vi "Dimostatore.vi"() -> ()   [LabVIEW 2019]
uses:
  ByteGSAPIBase.lvclass
  FetchCalibration/Converted_Slug_Cluster.ctl
  CalibrationMeasurements/BodyCalibrazioneMisure.ctl
  6d3d0a70-a223-4ddd-b0d3-7207305fe689.vi
  85eea304-0067-4311-882a-d02f57de18c2.vi
panel:
  out "Valore misurato":string
  out "Valore di riferimento":string
  in  "Start":bool
  in  "Send":bool
  out "Infobox":string
  out "Strumenti da calibrare":i32(listbox)
  in  "Exit":bool=TRUE
  in  "Calibrate":bool
  in  "error out":errorcluster
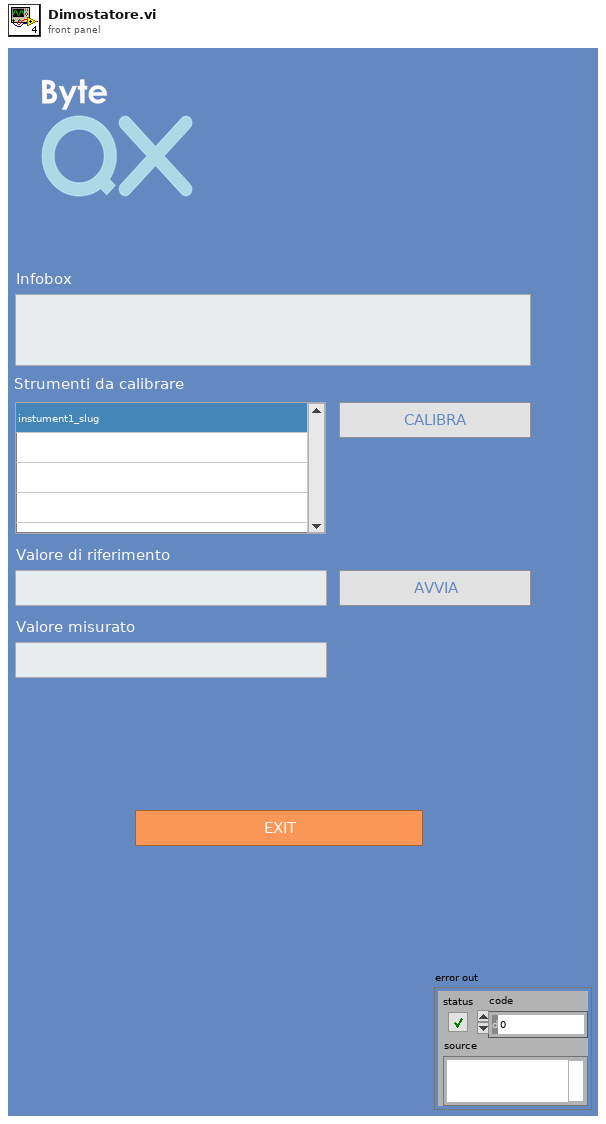
[diagram p1: front panel]
types:
  T1 = cluster{"nome":string, cluster{"Measurement_Id":i32, "Passed?":bool}[]}[]
  T2 = typedef "ByteGSWebAPI.lvlib/ByteGSAPIBase.lvclass/BodyCalibrazioneMisure.ctl" = cluster{"strumento_riferimento":cluster{"id":u16, "nome":string}, "controls":cluster{"id":u16, "descrizione":string, "numero_misure_necessarie":u16, "riferimento_obiettivo":dbl, "mpe_max":dbl, "mpe_min":dbl, "deviazione_standard":dbl, "incertezza":dbl}[], "temperatura_c":dbl, "umidita":dbl}
  T3 = typedef "ByteGSWebAPI.lvlib/ByteGSAPIBase.lvclass/Converted_Slug_Cluster.ctl" = cluster{"id":u32, "instrument":string, "name":string, "date":timestamp}
  T4 = cluster{"ByteGSAPIBase in":refnum<class "ByteGSAPIBase.lvclass">, "Expired_Instruments":T3[], "Calibrations":T2, "Strumenti_calibrati":cluster{"nome":string, cluster{"Measurement_Id":i32, "Passed?":bool}[]}[], "Instr_index":i32, "Calib_index":i32, "Instruments_Slug":string[]}
  T5 = cluster{"id":u16, "descrizione":string, "numero_misure_necessarie":u16, "riferimento_obiettivo":dbl, "mpe_max":dbl, "mpe_min":dbl, "deviazione_standard":dbl, "incertezza":dbl}[]
  T6 = cluster{"id":u16, "descrizione":string, "numero_misure_necessarie":u16, "riferimento_obiettivo":dbl, "mpe_max":dbl, "mpe_min":dbl, "deviazione_standard":dbl, "incertezza":dbl}
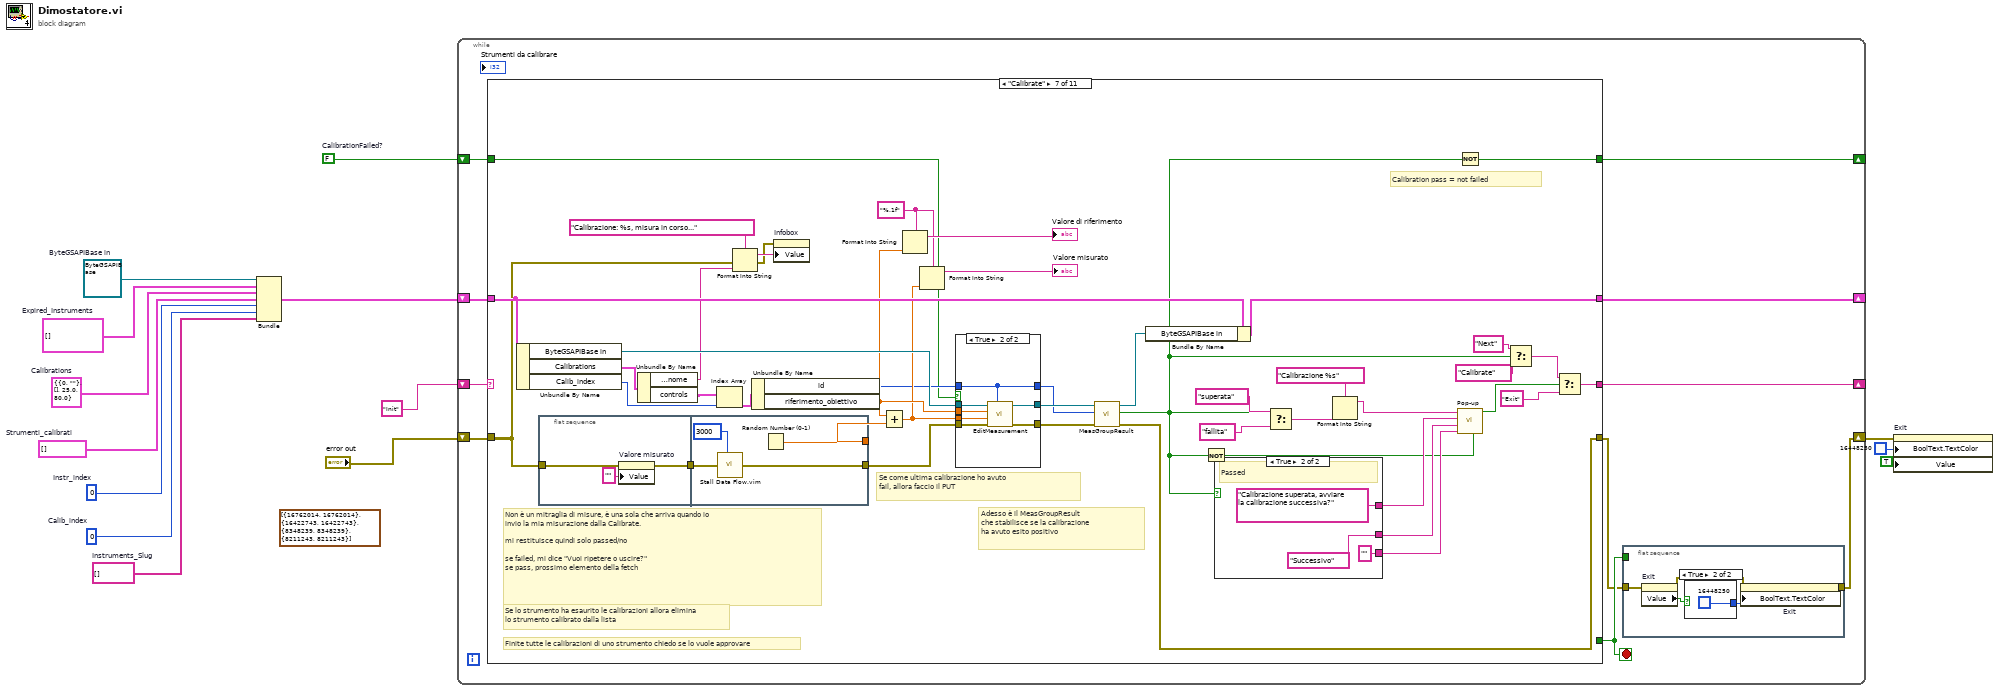
[diagram p0: block diagram]
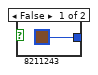
[diagram p2: hidden frame]
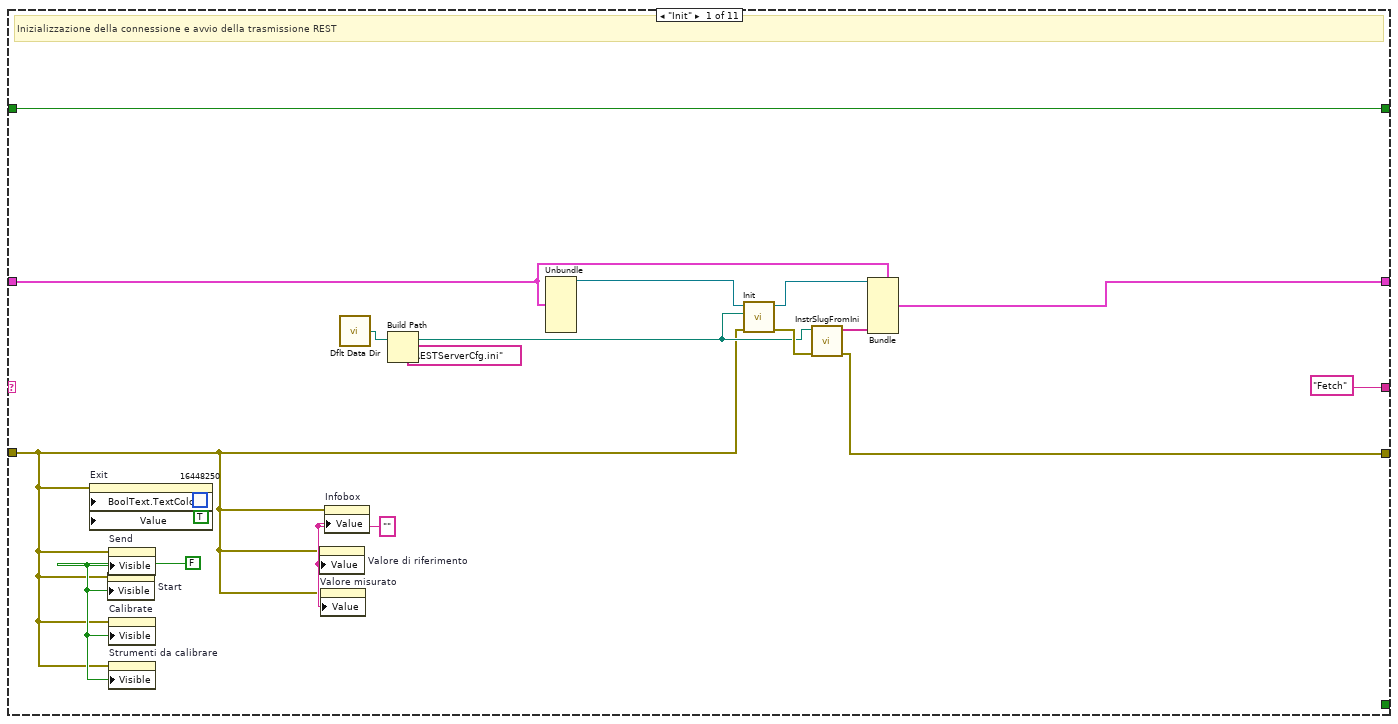
[diagram p3: hidden frame]
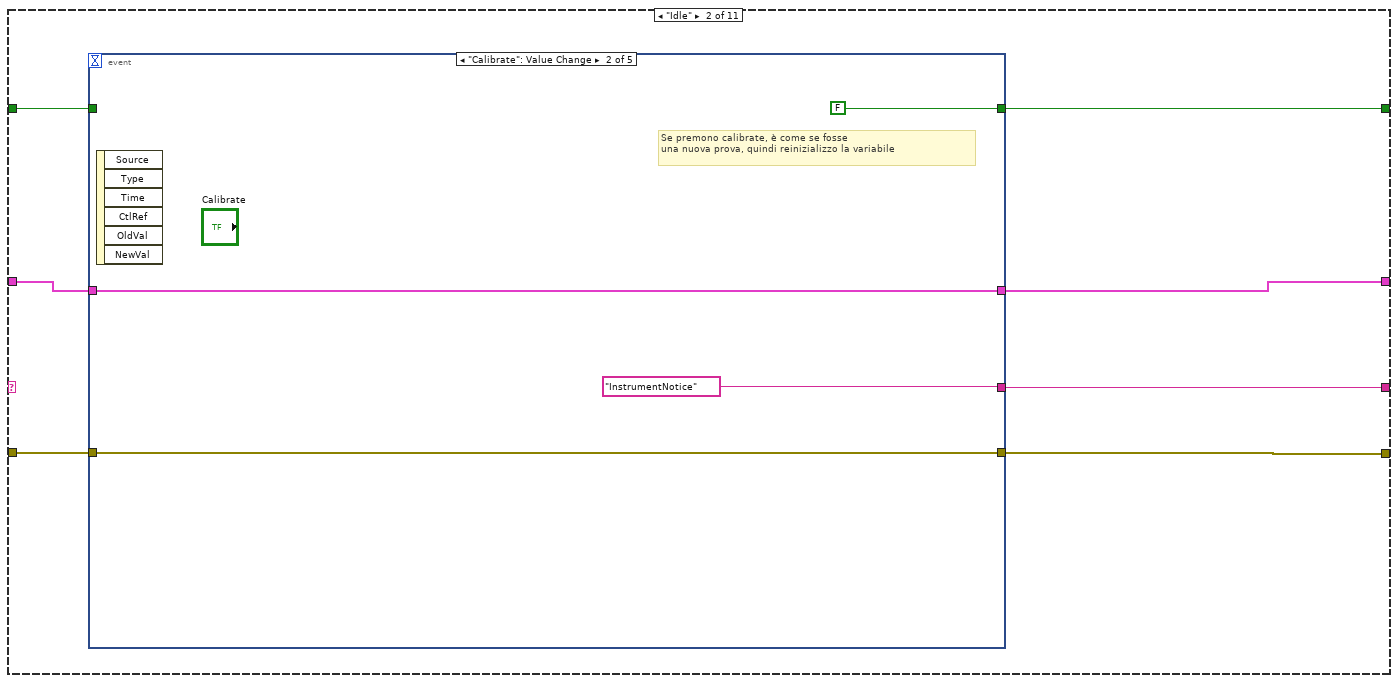
[diagram p4: hidden frame]
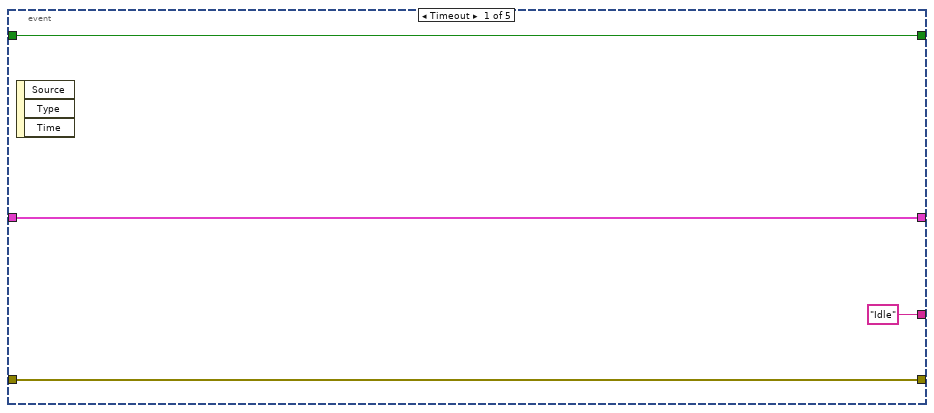
[diagram p5: hidden frame]
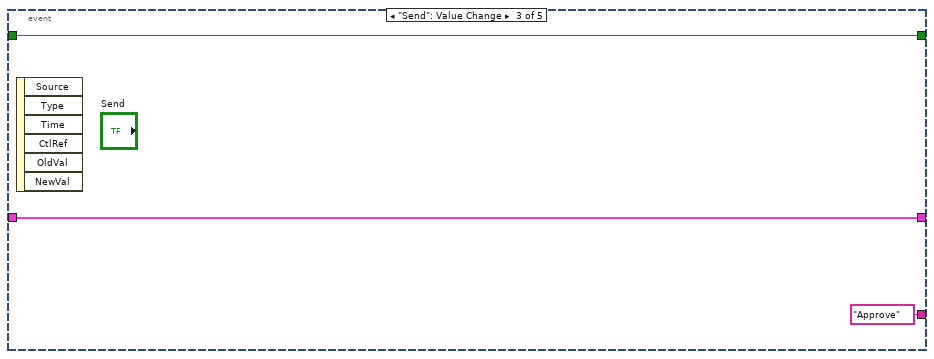
[diagram p6: hidden frame]
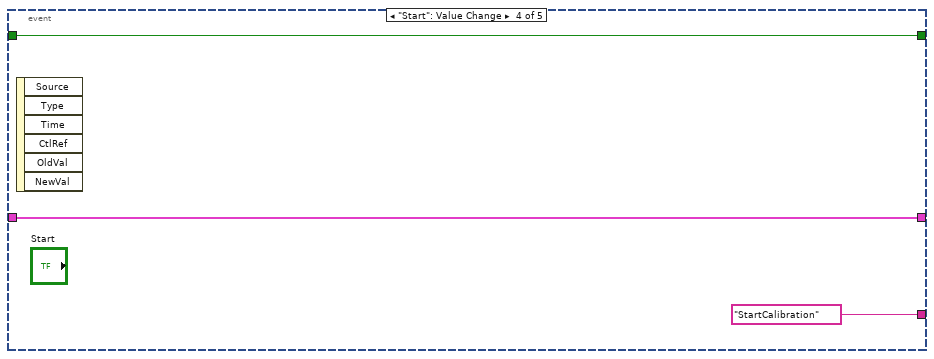
[diagram p7: hidden frame]
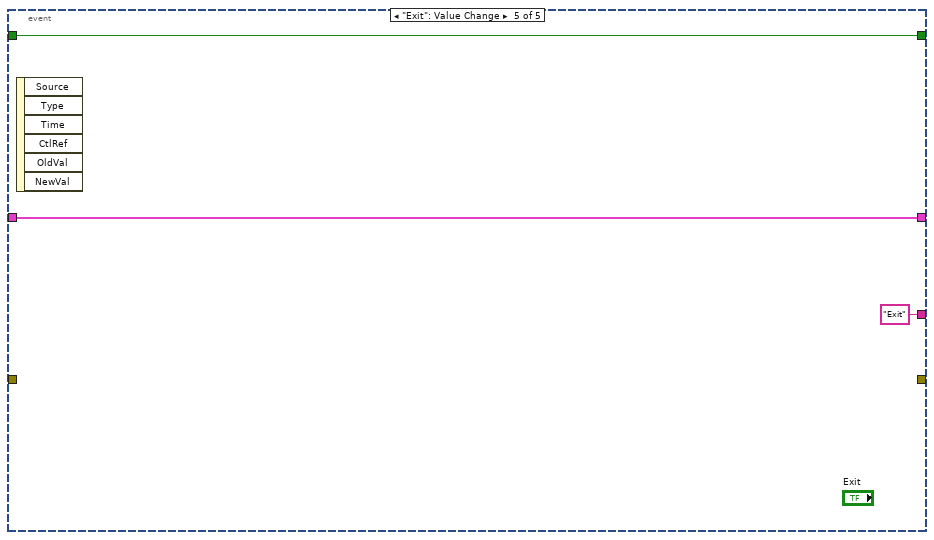
[diagram p8: hidden frame]
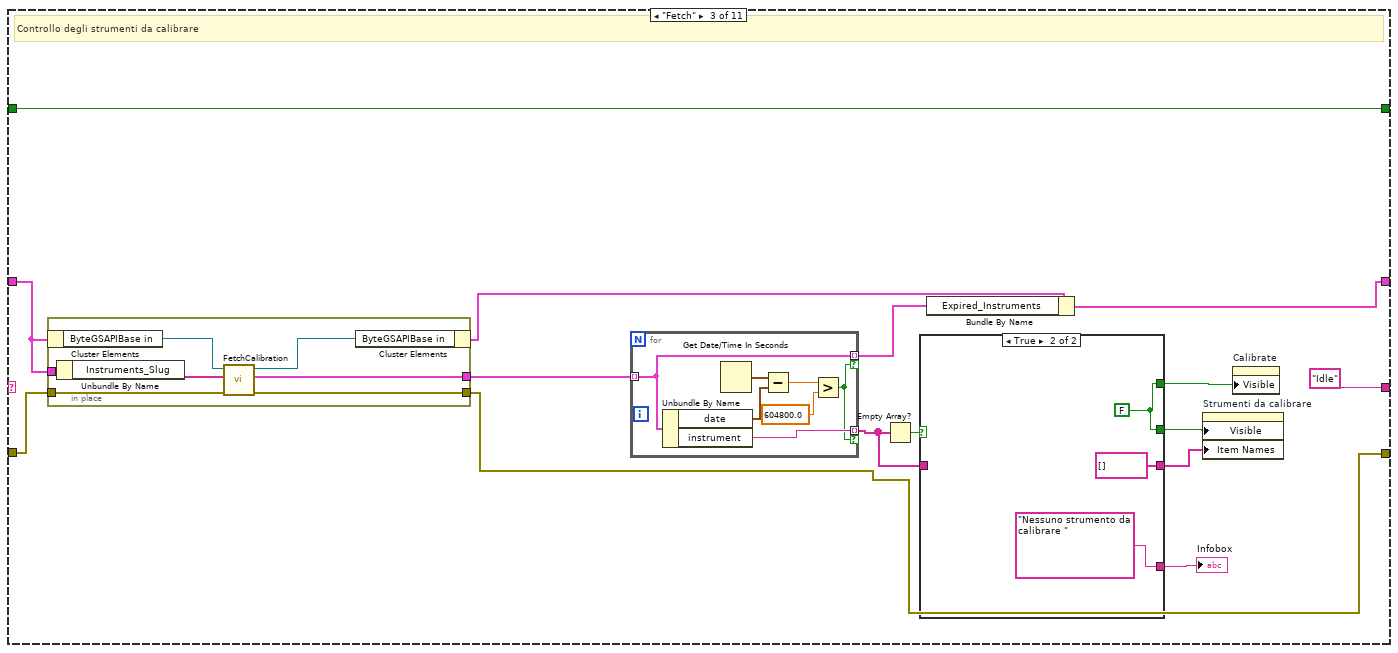
[diagram p9: hidden frame]
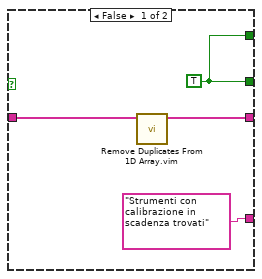
[diagram p10: hidden frame]
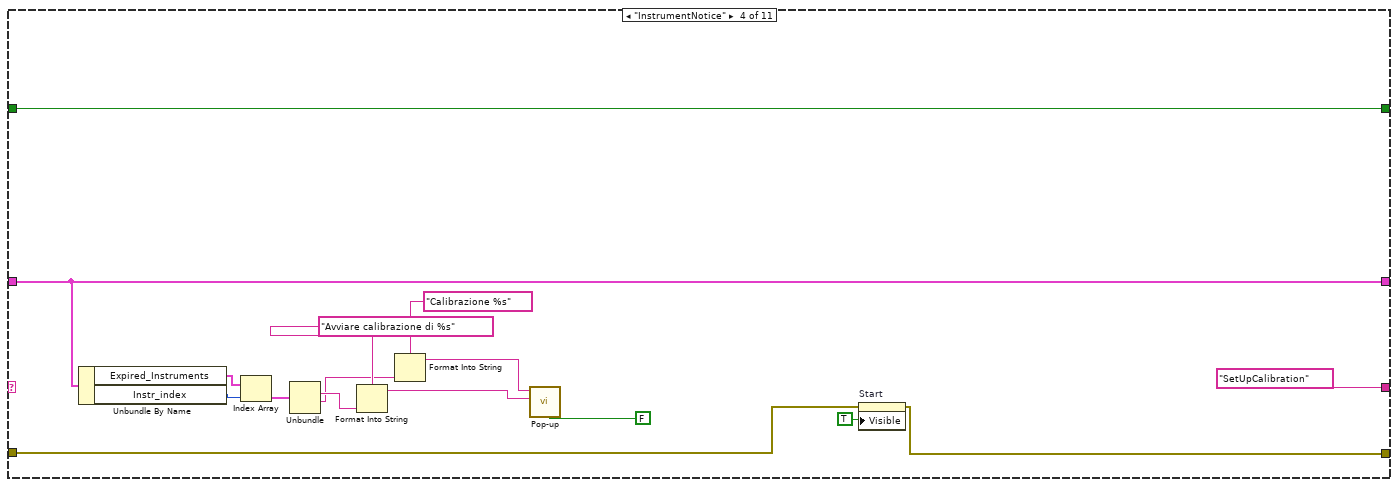
[diagram p11: hidden frame]
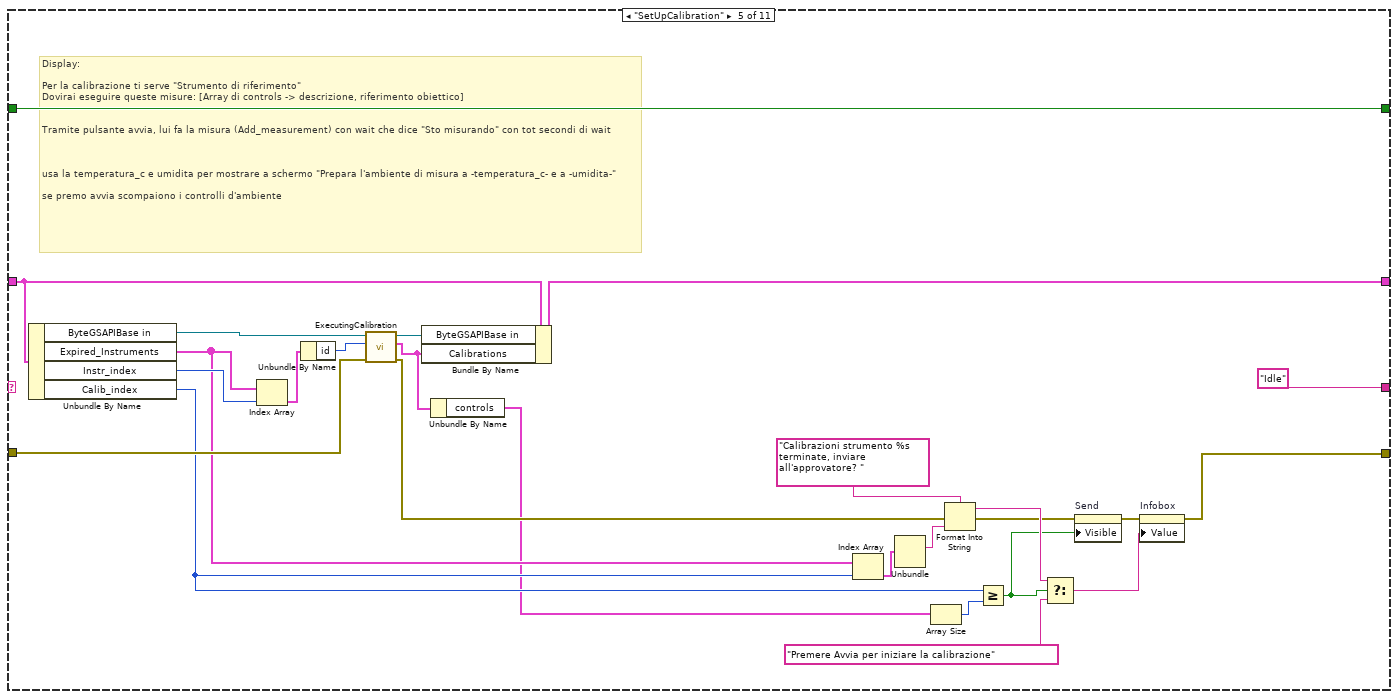
[diagram p12: hidden frame]
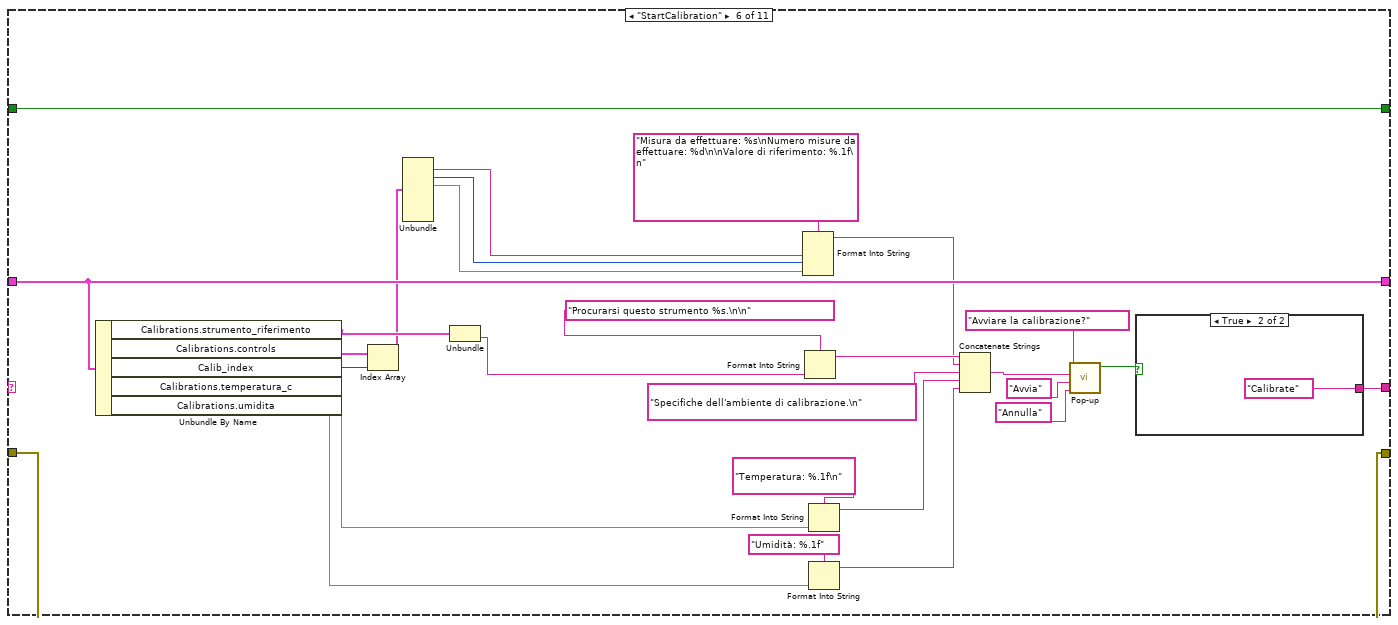
[diagram p13: hidden frame]
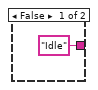
[diagram p14: hidden frame]
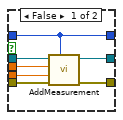
[diagram p15: hidden frame]
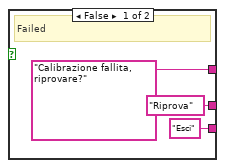
[diagram p16: hidden frame]
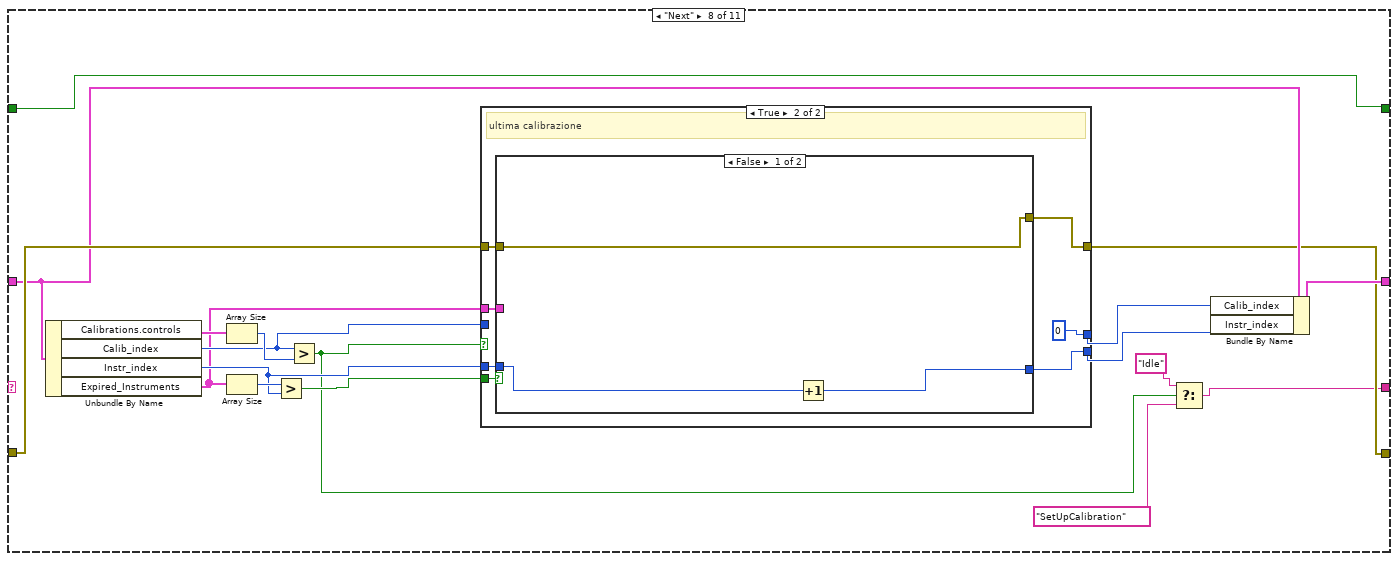
[diagram p17: hidden frame]
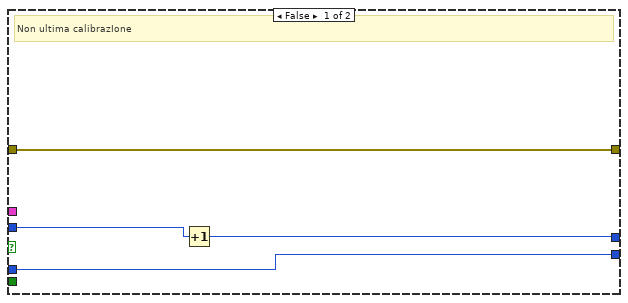
[diagram p18: hidden frame]
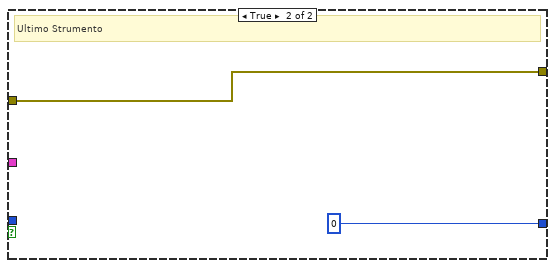
[diagram p19: hidden frame]
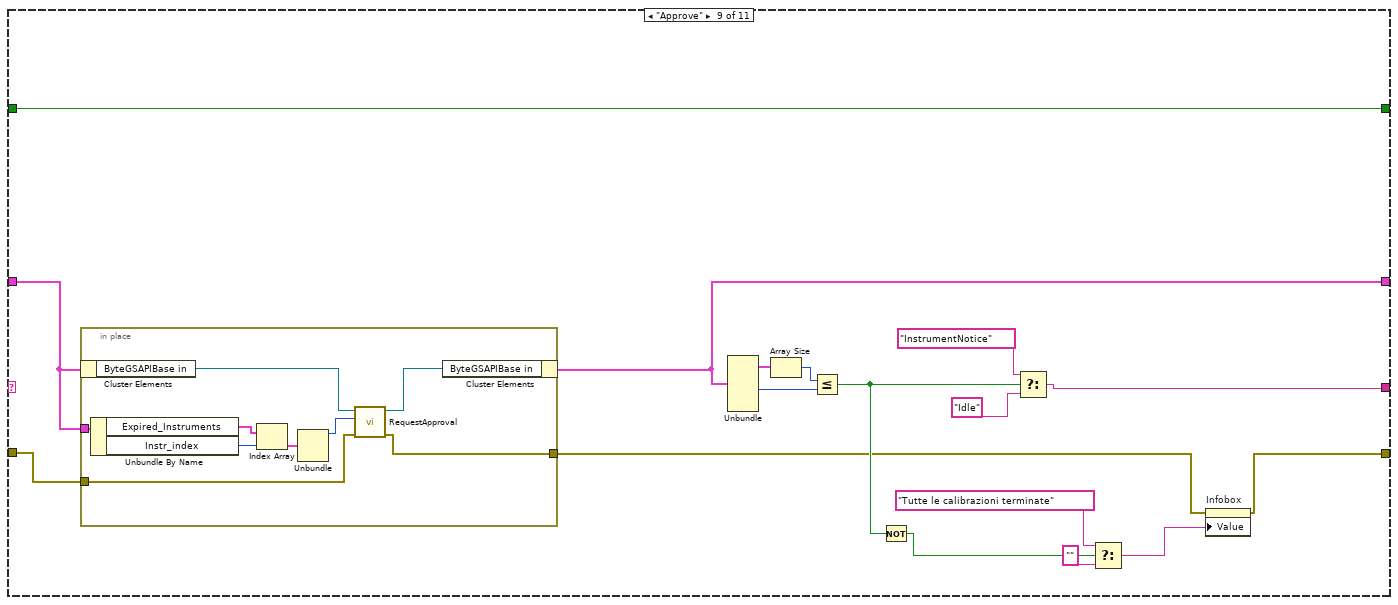
[diagram p20: hidden frame]
diagram:
  w1 = FALSE  # CalibrationFailed?
  w2 = string[] []  # Instruments_Slug
  w6 = 0  # Calib_index
  w7 = 0  # Instr_index
  w8 = T1 []  # Strumenti_calibrati
  w9 = T2 {"strumento_riferimento"={"id"=0, "nome"=""}, "controls"=[], "temperatura_c"=25.0, "umidita"=80.0}  # Calibrations
  (unwired) cluster{u32, u32}[] [{16762014, 16762014}, {16422743, 16422743}, {8348239, 8348239}, {8211243, 8211243}] ("Colors [4]")
  w10 = T3[] []  # Expired_Instruments
  w13 = refnum<class "ByteGSAPIBase.lvclass"> refnum  # ByteGSAPIBase in
  n1 = Bundle("ByteGSAPIBase in"=w13, "Expired_Instruments"=w10, "Calibrations"=w9, "Strumenti_calibrati"=w8, "Instr_index"=w7, "Calib_index"=w6, "Instruments_Slug"=w2) -> (w12:T4)  [unwired: 1 in]
  n2 = while {
    shift-right: [w21] -> _
    shift-left: w12 -> [w23]
    shift-right: [w17] -> w5
    shift-left: "error out" -> [w22]
    shift-right: [w20] -> _
    shift-left: "Init" -> [w24]
    shift-right: [w15] -> _
    shift-left: w1 -> [w16]
    stop <- w19 stop-if-true
    n3 = case shown="\"Calibrate\"" w24 {
      tunnel: w23 -> [w48 w52 w74 w124 w150 w178 w224 w261 w302 w315 w319]
      tunnel: w22 -> [w33 w54 w87 w112 w146 w168 w192 w262 w301 w316 w320]
      tunnel: [w36 w55 w75 w111 w141 w168 w188 w260 w287 w316 w320] -> w18
      tunnel: [w47 w53 w76 w124 w148 w178 w193 w268 w300 w315 w319] -> w21
      tunnel: [_ _ _ _ _ _ _ _ _ TRUE _] -> w19
      tunnel: ["Fetch" w51 "Idle" ("t") "SetUpCalibration" ("t") "Idle" ("t") w160 w199 w254 w294 "" ("t") "Exit" ("t")] -> w20
      tunnel: w16 -> [w32 w50 w73 w109 w125 w151 w183 w252 w286 w312 w317]
      tunnel: [w32 w49 w73 w109 w125 w151 w181 w252 w286 w312 w317] -> w15
      frame "Init" {
        w41 = "" ("Infobox")
        w40 = FALSE
        # "Inizializzazione della connessione e avvio della trasmissione REST"
        n4 = property on="Exit" class="Bool (strict)"(error in=w33, "BoolText.TextColor"=u32 16448250, "Value"=TRUE ("Exit")) -> ()  [unwired: 1 in, 2 out]
        n5 = property on="Start" class="Bool"(error in=w33, "Visible"=w40) -> ()  [unwired: 1 in, 2 out]
        n6 = property on="Send" class="Bool"(error in=w33, "Visible"=w40) -> ()  [unwired: 1 in, 2 out]
        n7 = property on="Calibrate" class="Bool"(error in=w33, "Visible"=w40) -> ()  [unwired: 1 in, 2 out]
        n8 = property on="Strumenti da calibrare" class="LstBox (strict)"(error in=w33, "Visible"=w40) -> ()  [unwired: 1 in, 2 out]
        n9 = property on="Valore di riferimento" class="Str"(error in=w33, "Value"=w41) -> ()  [unwired: 1 in, 2 out]
        n10 = property on="Valore misurato" class="Str"(error in=w33, "Value"=w41) -> ()  [unwired: 1 in, 2 out]
        n11 = property on="Infobox" class="Str"(error in=w33, "Value"=w41) -> ()  [unwired: 1 in, 2 out]
        n12 = call <vilib>:"Dflt Data Dir.vi"() -> ("App:Default Data Directory"=w39:path)
        n13 = Build Path(base path=w39, name or relative path="RESTServerCfg.ini") -> (appended path=w35:path)
        n14 = Unbundle(w48) -> ("ByteGSAPIBase in"=w43:refnum<class "ByteGSAPIBase.lvclass">)  [unwired: 6 out]
        n15 = call-dynamic "Init.vi"("error in (no error)"=w33, "configuration file path"=w35, "ByteGSAPIBase in"=w43) -> ("error out"=w37:errorcluster, "ByteGSAPIBase out"=w42:refnum<class "ByteGSAPIBase.lvclass">)  [unwired: 7 in]
        n16 = call "InstrSlugFromIni.vi"("error in (no error)"=w37, "configuration file path"=w35) -> ("error out"=w36:errorcluster, "Array"=w34:string[])  [unwired: 8 in]
        n17 = Bundle(cluster=w48, "ByteGSAPIBase in"=w42, "Instruments_Slug"=w34) -> (w47:T4)  [unwired: 5 in]
      }
      frame "Idle" {
        n18 = event shown="[1] \"Calibrate\": Value Change" {
          selector: _ -> [_ _ _ _ _]
          dyn-events: _ -> [_ _ _ _ _]
          timeout: _ -> [_ _ _ _ _]
          tunnel: [w59 w61 _ _ _] -> w55
          tunnel: w54 -> [w59 w61 _ _ _]
          tunnel: [w58 w63 w66 w69 w72] -> w53
          tunnel: w52 -> [w58 w63 w66 w69 w72]
          tunnel: ["Idle" ("t") "InstrumentNotice" "Approve" ("t") "StartCalibration" ("t") "Exit" ("t")] -> w51
          tunnel: w50 -> [w56 _ w64 w67 w70]
          tunnel: [w56 FALSE ("CalibrationFailed?") w64 w67 w70] -> w49
          event Timeout {
            n19 = event-data() -> ()  [unwired: 1 in, 3 out]
          }
          event "Calibrate": Value Change {
            # "Se premono calibrate, è come se fosse\nuna nuova prova, quindi reinizializzo la variabile"
            n20 = event-data() -> ()  [unwired: 1 in, 6 out]
          }
          event "Send": Value Change {
            n21 = event-data() -> ()  [unwired: 1 in, 6 out]
          }
          event "Start": Value Change {
            n22 = event-data() -> ()  [unwired: 1 in, 6 out]
          }
          event "Exit": Value Change {
            n23 = event-data() -> ()  [unwired: 1 in, 6 out]
          }
        }
      }
      frame "Fetch" {
        # "Controllo degli strumenti da calibrare"
        n24 = in-place {
          in-place-border: w87 -> [w93]
          in-place-border: [w92] -> w75
          in-place-border: [w91] -> w79
          in-place-border: w74 -> [w89]
          n25 = in-place-cluster #1(w74) -> ("ByteGSAPIBase in"=w90:refnum<class "ByteGSAPIBase.lvclass">)
          n26 = Unbundle By Name(w89) -> ("Instruments_Slug"=w88:string[])
          n27 = call "FetchCalibration.vi"("error in (no error)"=w93, "Instruments"=w88, "ByteGSAPIBase in"=w90) -> ("error out"=w92:errorcluster, "Instruments"=w91:T3[], "ByteGSAPIBase out"=w94:refnum<class "ByteGSAPIBase.lvclass">)  [unwired: 6 in]
          n28 = in-place-cluster #1("ByteGSAPIBase in"=w94) -> (w86:T4)
        }
        n29 = for {
          tunnel: w79 -> [w97] mode=indexing
          tunnel: [w97] -> w78 mode=indexing if=w95
          tunnel: [w96] -> w84 mode=indexing if=w95
          n30 = Unbundle By Name(w97) -> ("date"=w98:timestamp, "instrument"=w96:string)
          n31 = Get Date/Time In Seconds() -> (seconds since 1Jan1904=w100:timestamp)
          n32 = Subtract(x=w100, y=w98) -> (x-y=w101:dbl)
          n33 = Greater?(x=w101, y=604800.0) -> (0:w95:bool)
        }
        n34 = Empty Array?(array=w84) -> (empty?=w85:bool)
        n35 = case shown="True" w85 {
          tunnel: w84 -> [w104 _]
          tunnel: [w102 w106] -> w83
          tunnel: ["Strumenti con calibrazione in scadenza trovati" ("Infobox") "Nessuno strumento da calibrare " ("Infobox")] -> w82
          tunnel: [w103 string[] []] -> w81
          tunnel: [w102 w106] -> w77
          frame False {
            w102 = TRUE ("Visible")
            n36 = call "Remove Duplicates From 1D Array.vim"("array"=w104) -> ("array with duplicates removed"=w103:string[])  [unwired: 10 in]
          }
          frame True {
            w106 = FALSE ("Visible")
          }
        }
        "Infobox" <- w82
        n37 = Bundle By Name(cluster=w86, "Expired_Instruments"=w78) -> (w76:T4)
        n38 = property on="Strumenti da calibrare" class="LstBox (strict)"("Visible"=w83, "Item Names"=w81) -> ()  [unwired: 2 in, 2 out]
        n39 = property on="Calibrate" class="Bool"("Visible"=w77) -> ()  [unwired: 2 in, 2 out]
      }
      frame "InstrumentNotice" {
        n40 = Unbundle By Name(w124) -> ("Expired_Instruments"=w123:T3[], "Instr_index"=w122:i32)
        n41 = Index Array(array=w123, index=w122) -> (element=w121:T3)
        n42 = Unbundle(w121) -> ("instrument"=w119:string, "name"=w117:string)  [unwired: 2 out]
        n43 = Format Into String(format string="Avviare calibrazione di %s" ("Title"), w119) -> (resulting string=w118:string)  [unwired: 2 in, 1 out]
        n44 = Format Into String(format string="Calibrazione %s", w117) -> (resulting string=w115:string)  [unwired: 2 in, 1 out]
        n45 = call "Pop-up.vi"("Two_btn"=FALSE, "Text"=w118, "Title"=w115) -> ()  [unwired: 8 in, 1 out]
        n46 = property on="Start" class="Bool"(error in=w112, "Visible"=TRUE) -> (error out=w111:errorcluster)  [unwired: 1 in, 1 out]
      }
      frame "SetUpCalibration" {
        # "Display: \n\nPer la calibrazione ti serve \"Strumento di riferimento\"\nDovirai eseguire queste misure: [Array di controls -> descrizione, riferimento obiettico] \n\n\nTramite pulsante avvia, lui fa la misura (Add_measurement) con wait che dice \"Sto misurando\" con tot secondi di wait\n\n\n\nusa la temperatura_c e umidita per mostrare a schermo \"Prepara l'ambiente di misura a -temperatura_c- e a -umidita-\"\n\nse premo avvia scompaiono i controlli d'ambiente"
        n47 = Unbundle By Name(w150) -> ("ByteGSAPIBase in"=w149:refnum<class "ByteGSAPIBase.lvclass">, "Expired_Instruments"=w137:T3[], "Instr_index"=w142:i32, "Calib_index"=w135:i32)
        n48 = Index Array(array=w137, index=w142) -> (element=w143:T3)
        n49 = Unbundle By Name(w143) -> ("id"=w144:u32)
        n50 = call "ExecutingCalibration.vi"("error in (no error)"=w146, "calibration_id"=w144, "ByteGSAPIBase in"=w149) -> ("error out"=w130:errorcluster, "Cluster"=w127:T2, "ByteGSAPIBase out"=w147:refnum<class "ByteGSAPIBase.lvclass">)  [unwired: 6 in]
        n51 = Bundle By Name(cluster=w150, "ByteGSAPIBase in"=w147, "Calibrations"=w127) -> (w148:T4)
        n52 = Unbundle By Name(w127) -> ("controls"=w126:T5)
        n53 = Index Array(array=w137, index=w135) -> (element=w138:T3)
        n54 = Unbundle(w138) -> ("instrument"=w136:string)  [unwired: 3 out]
        n55 = Array Size(array=w126) -> (size(s)=w134:i32)
        n56 = Format Into String(format string="Calibrazioni strumento %s terminate, inviare all'approvatore? ", error in=w130, w136) -> (resulting string=w140:string, error out=w129:errorcluster)  [unwired: 1 in]
        n57 = Greater Or Equal?(x=w135, y=w134) -> (x >= y?=w131:bool)
        n58 = Select(t=w140, s=w131, f="Premere Avvia per iniziare la calibrazione" ("Infobox")) -> (s? t:f=w132:string)
        n59 = property on="Send" class="Bool"(error in=w129, "Visible"=w131) -> (error out=w128:errorcluster)  [unwired: 1 in, 1 out]
        n60 = property on="Infobox" class="Str"(error in=w128, "Value"=w132) -> (error out=w141:errorcluster)  [unwired: 1 in, 1 out]
      }
      frame "StartCalibration" {
        n61 = Unbundle By Name(w178) -> ("Calibrations.strumento_riferimento"=w173:cluster{"id":u16, "nome":string}, "Calibrations.controls"=w158:T5, "Calib_index"=w159:i32, "Calibrations.temperatura_c"=w162:dbl, "Calibrations.umidita"=w163:dbl)
        n62 = Index Array(array=w158, index=w159) -> (element=w157:T6)
        n63 = Unbundle(w157) -> ("descrizione"=w155:string, "numero_misure_necessarie"=w152:u16, "riferimento_obiettivo"=w153:dbl)  [unwired: 5 out]
        n64 = Unbundle(w173) -> ("nome"=w170:string)  [unwired: 1 out]
        n65 = Format Into String(format string="Misura da effettuare: %s\nNumero misure da effettuare: %d\n\nValore di riferimento: %.1f\n", w155, w152, w153) -> (resulting string=w156:string)  [unwired: 2 in, 1 out]
        n66 = Format Into String(format string="Procurarsi questo strumento %s.\n\n", w170) -> (resulting string=w177:string)  [unwired: 2 in, 1 out]
        n67 = Format Into String(format string="Temperatura: %.1f\n", w162) -> (resulting string=w167:string)  [unwired: 2 in, 1 out]
        n68 = Format Into String(format string="Umidità: %.1f", w163) -> (resulting string=w165:string)  [unwired: 2 in, 1 out]
        n69 = Concatenate Strings(w177, w156, "Specifiche dell'ambiente di calibrazione.\n" ("string"), w167, w165) -> (w171:string)
        n70 = call "Pop-up.vi"("CancelText"="Annulla", "OkText"="Avvia", "Text"=w171, "Title"="Avviare la calibrazione?") -> ("Btn-OK Out"=w161:bool)  [unwired: 7 in]
        n71 = case shown="True" w161 {
          tunnel: ["Idle" "Calibrate"] -> w160
          frame False {
          }
          frame True {
          }
        }
      }
      frame "Calibrate" {
        w212 = "%.1f" ("format string")
        # "Calibration pass = not failed"
        # "Se come ultima calibrazione ho avuto\nfail, allora faccio il PUT"
        # "Adesso è il MeasGroupResult\nche stabilisce se la calibrazione\nha avuto esito positivo"
        # "Finite tutte le calibrazioni di uno strumento chiedo se lo vuole approvare"
        # "Se lo strumento ha esaurito le calibrazioni allora elimina\nlo strumento calibrato dalla lista"
        # "Non è un mitraglia di misure, è una sola che arriva quando io\ninvio la mia misurazione dalla Calibrate.\n\nmi restituisce quindi solo passed/no \n\nse failed, mi dice \"Vuoi ripetere o uscire?\"\nse pass, prossimo elemento della fetch"
        n72 = Unbundle By Name(w224) -> ("ByteGSAPIBase in"=w223:refnum<class "ByteGSAPIBase.lvclass">, "Calibrations"=w222:T2, "Calib_index"=w215:i32)
        n73 = flat-sequence {
          tunnel: w192 -> [w240]
          tunnel: [w241] -> w190
          tunnel: [w245] -> w210
          tunnel: [w242] -> w191
          tunnel: w190 -> [w243]
          frame #0 {
            n74 = property on="Valore misurato" class="Str"(error in=w240, "Value"="" ("Valore misurato")) -> (error out=w241:errorcluster)  [unwired: 1 in, 1 out]
          }
          frame #1 {
            n75 = call "Stall Data Flow.vim"("value in"=w243, "milliseconds to wait"=u32 3000) -> ("value out"=w242:errorcluster)  [unwired: 1 out]
            n76 = Random Number (0-1)() -> (number: 0 to 1=w245:dbl)
          }
        }
        n77 = Unbundle By Name(w222) -> ("strumento_riferimento.nome"=w218:string, "controls"=w216:T5)
        n78 = Index Array(array=w216, index=w215) -> (element=w217:T6)
        n79 = Format Into String(format string="Calibrazione: %s, misura in corso...", error in=w192, w218) -> (resulting string=w221:string, error out=w220:errorcluster)  [unwired: 1 in]
        n80 = Unbundle By Name(w217) -> ("id"=w187:u16, "riferimento_obiettivo"=w214:dbl)
        n81 = property on="Infobox" class="Str"(error in=w220, "Value"=w221) -> ()  [unwired: 1 in, 2 out]
        n82 = Add(x=w214, y=w210) -> (x+y=w194:dbl)
        n83 = Format Into String(format string=w212, w214) -> (resulting string=→"Valore di riferimento":string)  [unwired: 2 in, 1 out]
        n84 = Format Into String(format string=w212, w194) -> (resulting string=→"Valore misurato":string)  [unwired: 2 in, 1 out]
        n85 = case shown="True" w183 {
          tunnel: w223 -> [w231 w238]
          tunnel: w214 -> [w230 w236]
          tunnel: w194 -> [w229 w235]
          tunnel: w191 -> [w228 w237]
          tunnel: [w227 w232] -> w189
          tunnel: w187 -> [w225 w234]
          tunnel: [w226 w233] -> w186
          tunnel: [w225 w234] -> w184
          frame False {
            n86 = call-dynamic "AddMeasurement.vi"("measurement_group id"=w225, "error in (no error)"=w228, "misura_strumento"=w229, "misura_riferimento"=w230, "ByteGSAPIBase in"=w231) -> ("error out"=w227:errorcluster, "ByteGSAPIBase out"=w226:refnum<class "ByteGSAPIBase.lvclass">)  [unwired: 3 in, 2 out]
          }
          frame True {
            n87 = call-dynamic "EditMeasurement.vi"("measurement_group id"=w234, "error in (no error)"=w237, "misura_strumento"=w235, "misura_riferimento"=w236, "ByteGSAPIBase in"=w238) -> ("error out"=w232:errorcluster, "ByteGSAPIBase out"=w233:refnum<class "ByteGSAPIBase.lvclass">)  [unwired: 3 in, 2 out]
          }
        }
        n88 = call "MeasGroupResult.vi"("error in (no error)"=w189, "measurement_group_id"=w184, "ByteGSAPIBase in"=w186) -> ("error out"=w188:errorcluster, "measurement_group_passed"=w182:bool, "ByteGSAPIBase out"=w185:refnum<class "ByteGSAPIBase.lvclass">)  [unwired: 5 in, 1 out]
        n89 = Bundle By Name(cluster=w224, "ByteGSAPIBase in"=w185) -> (w193:T4)
        n90 = Not(x=w182) -> (.not. x?=w198:bool)
        n91 = case shown="True" w182 {
          tunnel: ["Riprova" "Successivo"] -> w204
          tunnel: ["Esci" ""] -> w203
          tunnel: ["Calibrazione fallita, riprovare?" ("Text") "Calibrazione superata, avviare la calibrazione successiva?" ("Text")] -> w202
          frame False {
            # "Failed"
          }
          frame True {
            # "Passed"
          }
        }
        n92 = Select(t="superata", s=w182, f="fallita") -> (s? t:f=w208:string)
        n93 = Format Into String(format string="Calibrazione %s", w208) -> (resulting string=w205:string)  [unwired: 2 in, 1 out]
        n94 = Not(x=w182) -> (.not. x?=w181:bool)
        n95 = call "Pop-up.vi"("Two_btn"=w198, "CancelText"=w203, "OkText"=w204, "Text"=w202, "Title"=w205) -> ("Btn-OK Out"=w201:bool)  [unwired: 6 in]
        n96 = Select(t="Next", s=w182, f="Calibrate") -> (s? t:f=w196:string)
        n97 = Select(t=w196, s=w201, f="Exit") -> (s? t:f=w199:string)
      }
      frame "Next" {
        n98 = Unbundle By Name(w261) -> ("Calibrations.controls"=w259:T5, "Calib_index"=w264:i32, "Instr_index"=w263:i32, "Expired_Instruments"=w258:T3[])
        n99 = Array Size(array=w259) -> (size(s)=w269:i32)
        n100 = Array Size(array=w258) -> (size(s)=w266:i32)
        n101 = Greater?(x=w266, y=w263) -> (0:w257:bool)
        n102 = Greater?(x=w264, y=w269) -> (0:w253:bool)
        n103 = case shown="True" w253 {
          tunnel: [w272 0 ("Calib_index")] -> w267
          tunnel: w264 -> [w273 _]
          tunnel: w263 -> [w271 w278]
          tunnel: w257 -> [_ w280]
          tunnel: [w271 w277] -> w265
          tunnel: w262 -> [w270 w276]
          tunnel: [w270 w275] -> w260
          tunnel: w258 -> [_ w274]
          frame False {
            # "Non ultima calibrazIone"
            n104 = Increment(x=w273) -> (x+1=w272:i32)
          }
          frame True {
            # "ultima calibrazione"
            n105 = case shown="False" w280 {
              tunnel: w278 -> [w283 _]
              tunnel: [w282 0] -> w277
              tunnel: w276 -> [w281 w284]
              tunnel: [w281 w284] -> w275
              tunnel: w274 -> [_ _]
              frame False {
                n106 = Increment(x=w283) -> (x+1=w282:i32)
              }
              frame True {
                # "Ultimo Strumento"
              }
            }
          }
        }
        n107 = Select(t="Idle", s=w253, f="SetUpCalibration") -> (s? t:f=w254:string)
        n108 = Bundle By Name(cluster=w261, "Calib_index"=w267, "Instr_index"=w265) -> (w268:T4)
      }
      frame "Approve" {
        n109 = in-place {
          in-place-border: w302 -> [w309]
          in-place-border: w301 -> [w308]
          in-place-border: [w307] -> w288
          n110 = in-place-cluster #2(w302) -> ("ByteGSAPIBase in"=w311:refnum<class "ByteGSAPIBase.lvclass">)
          n111 = Unbundle By Name(w309) -> ("Expired_Instruments"=w306:T3[], "Instr_index"=w305:i32)
          n112 = Index Array(array=w306, index=w305) -> (element=w304:T3)
          n113 = Unbundle(w304) -> ("id"=w303:u32)  [unwired: 3 out]
          n114 = call "RequestApproval.vi"("error in (no error)"=w308, "calibration_id"=w303, "ByteGSAPIBase in"=w311) -> ("error out"=w307:errorcluster, "ByteGSAPIBase out"=w310:refnum<class "ByteGSAPIBase.lvclass">)  [unwired: 6 in, 1 out]
          n115 = in-place-cluster #2("ByteGSAPIBase in"=w310) -> (w300:T4)
        }
        n116 = Unbundle(w300) -> ("Expired_Instruments"=w299:T3[], "Instr_index"=w297:i32)  [unwired: 5 out]
        n117 = Array Size(array=w299) -> (size(s)=w298:i32)
        n118 = Less Or Equal?(x=w298, y=w297) -> (x <= y?=w291:bool)
        n119 = Not(x=w291) -> (.not. x?=w290:bool)
        n120 = Select(t="InstrumentNotice", s=w291, f="Idle") -> (s? t:f=w294:string)
        n121 = Select(t="Tutte le calibrazioni terminate", s=w290, f="") -> (s? t:f=w289:string)
        n122 = property on="Infobox" class="Str"(error in=w288, "Value"=w289) -> (error out=w287:errorcluster)  [unwired: 1 in, 1 out]
      }
      frame "Exit" {
        # "Uscita"
      }
      frame Default {
        # "Qua non dovrebbe entrarci"
      }
    }
    n123 = flat-sequence {
      tunnel: w19 -> [_]
      tunnel: [w27] -> w17
      tunnel: w18 -> [w26]
      frame #0 {
        n124 = property on="Exit" class="Bool (strict)"(error in=w26) -> (error out=w25:errorcluster, "Value"=w28:bool)  [unwired: 1 in, 1 out]
        n125 = case shown="True" w28 {
          tunnel: [u32 8211243 u32 16448250 ("Boolean Text.Text Colors:Text Color")] -> w29
          frame False {
          }
          frame True {
          }
        }
        n126 = property on="Exit" class="Bool (strict)"(error in=w25, "BoolText.TextColor"=w29) -> (error out=w27:errorcluster)  [unwired: 1 in, 1 out]
      }
    }
  }
  n127 = property on="Exit" class="Bool (strict)"(error in=w5, "BoolText.TextColor"=u32 16448250 ("Boolean Text.Text Colors:Text Color"), "Value"=TRUE ("Exit")) -> ()  [unwired: 1 in, 2 out]
